vi "Read ChassisType.vi"(8 "error in (no error)":errorcluster, 11 "Chassis BOM in":refnum<class "Chassis BOM.lvclass">) -> (0 "error out":errorcluster, 2 "ChassisType":T1, 3 "Chassis BOM out":refnum<class "Chassis BOM.lvclass">)   [LabVIEW 2012, in "Configuration Grandmaster.lvlib" / "Chassis BOM.lvclass"]
uses:
  Chassis BOM.lvclass
  Common/Controls/Chassis Type.ctl
  Chassis BOM.lvclass/Chassis BOM.ctl
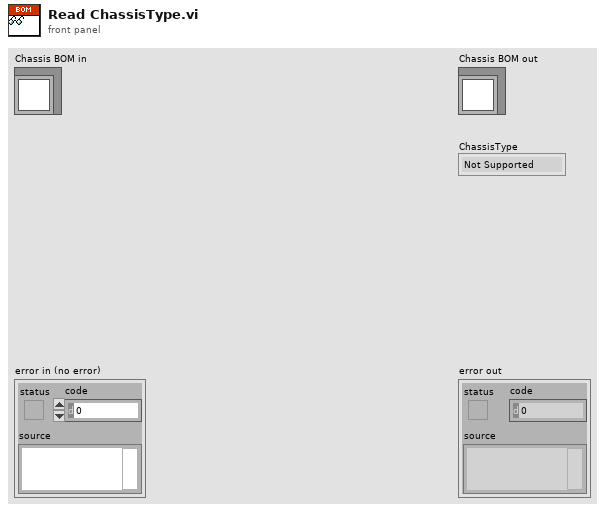
[diagram p1: front panel]
types:
  T1 = typedef "Chassis Type.ctl" = enum16{"Not Supported", "C Series 1-Slot", "C Series 4-Slot", "C Series 8-Slot", "PXI 8-Slot", "PXIe 18-Slot"}
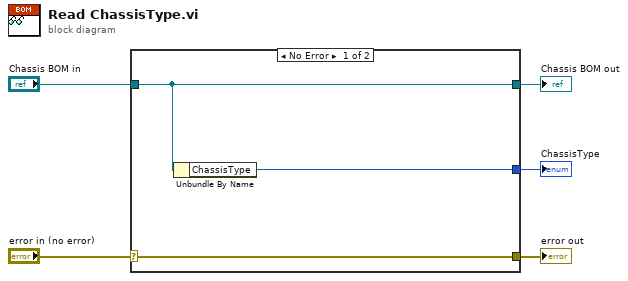
[diagram p0: block diagram]
diagram:
  n1 = case shown="No Error" "error in (no error)" {
    selector: "error in (no error)" -> [w8 w9]
    tunnel: [w8 w9] -> w4
    tunnel: [w7 w10] -> w2
    tunnel: "Chassis BOM in" -> [w7 w10]
    tunnel: [w6 _] -> w1
    frame No Error {
      n2 = Unbundle By Name(w7) -> ("ChassisType"=w6:T1)
    }
    frame Error {
    }
  }
  "error out" <- w4
  "Chassis BOM out" <- w2
  "ChassisType" <- w1
